vi "Inject Teller Metadata.vi"(4 "Priority":bool, 7 "Actor in":refnum<class "Actor.lvclass">, 8 "Error in":errorcluster, 9 "Reply":bool, 10 "Msg":refnum<class "Msg.lvclass">) -> (2 "Teller Metadata":refnum<class "Teller Metadata.lvclass">)   [LabVIEW 2020, in "jettl.lvlib"]
uses:
  jettl.lvlib
  Actor/Actor.lvclass
  Teller Metadata/Teller Metadata.lvclass
  Msg/Msg.lvclass
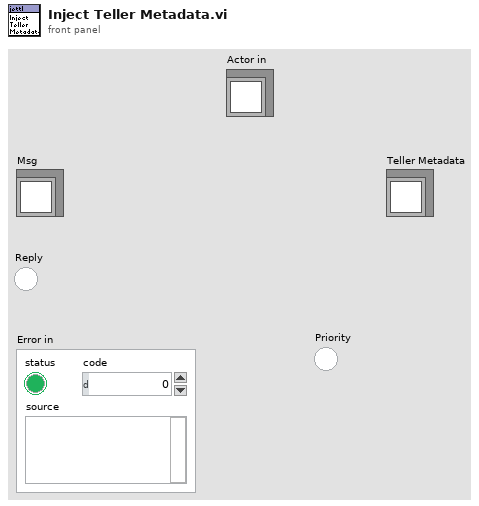
[diagram p1: front panel]
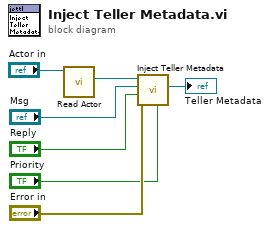
[diagram p0: block diagram]
diagram:
  n1 = call-dynamic "Read Actor.vi"("Actor in"="Actor in") -> ("Actor"=w6:refnum<class "Actor.lvclass">)  [unwired: 10 in]
  n2 = call-dynamic "Inject Teller Metadata.vi"("Priority"="Priority", "Error in"="Error in", "Reply"="Reply", "Msg"="Msg", "Actor in"=w6) -> ("Teller Metadata"=→"Teller Metadata":refnum<class "Teller Metadata.lvclass">)  [unwired: 6 in]
